vi "HEWH_WT300.vi"(4 "Manual Range (20 <10> A)":dbl(ring)=0.025 items=["5m <2.5m>"=0.0025, "10m <5m>"=0.005, "20m <10m>"=0.01, "50m <25m>"=0.025, "100m <50m>"=0.05, "200m <100m>"=0.1, "500m <250m>"=0.25, "1 <500m>"=0.5, "2 <1>"=1.0, "5 <2.5>"=2.5, "10 <5>"=5.0, "20 <10>"=10.0, "40 <20>"=20.0], 6 "Range Configuration (True)":bool[](array[boolean])=[FALSE, FALSE, FALSE, TRUE, FALSE, FALSE, FALSE, FALSE, FALSE, FALSE, FALSE, FALSE, FALSE], 8 "error in":errorcluster, 9 "Enable Auto Range (F: Disable)":bool, 11 "Message Queues out":T2) -> (0 "error out":errorcluster)   [LabVIEW 2023]
uses:
  Tenney/support/Message Queue/All Message Queues.ctl
  Tenney/support/Message Queue/Message Cluster.ctl
  Utility/Type Definitions/UTILITY Power Data.ctl
  Utility/Type Definitions/UTILITY Notifier.ctl
  FVIR and LDO/support/Message Queue/Enqueue Message (Single).vi
  FVIR and LDO/support/Message Queue/Message Queue.lvlib
  Drivers/Yokogawa WT300 Series/Yokogawa WT300 Series.lvlib
  Tenney/support/Message Queue/Tenney Message Queue.lvlib
panel:
  out "Loop Count":i32
  out "Power Data":T1={"Current (A):Element 1"=236.2, "Current (A):Element 2"=17.749, "Power (W):Sigma"=4192.0, "Watt Hours (Wh):Sigma"=0.0, "Voltage (V):Element 2"=236.2, "Voltage (V):Element 1"=236.2, "Current Crest Factor:Element 1"=0.0, "Current Crest Factor:Element 2"=0.0, "Voltage Harmonic (%):Element 1"=0.0, "Voltage Harmonic (%):Element 2"=0.0, "Voltage Crest Factor:Element 1"=0.0, "Voltage Crest Factor:Element 2"=0.0, "Time:Element 1"=0.0, "Frequency (Hz):Element 1"=0.0, "Apparent Power (VA):Element 1"=0.0, "Apparent Power (VA):Element 2"=0.0, "Power Factor:Element 1"=0.0, "Power Factor:Element 2"=0.0, "Max Watt Hours"=0.0, "Voltage (V):Element 2 Avg"=0.0, "Voltage (V):Element 1 Avg"=0.0} {"Voltage (V):Element 1 Avg" format="%.3g"; "Voltage (V):Element 2 Avg" format="%.3g"; "Max Watt Hours" format="%.3g"; "Power Factor:Element 2" format="%.3g"; "Power Factor:Element 1" format="%.3g"; "Apparent Power (VA):Element 2" format="%.3g"; "Apparent Power (VA):Element 1" format="%.3g"; "Frequency (Hz):Element 1" format="%.3g"; "Time:Element 1" format="%.3g"; "Voltage Crest Factor:Element 2" format="%.3g"; "Voltage Crest Factor:Element 1" format="%.3g"; "Voltage Harmonic (%):Element 2" format="%.3g"; "Voltage Harmonic (%):Element 1" format="%.3g"; "Current Crest Factor:Element 2" format="%.3g"; "Current Crest Factor:Element 1" format="%.3g"; "Voltage (V):Element 1" format="%.3g"; "Voltage (V):Element 2" format="%.3g"; "Watt Hours (Wh):Sigma" format="%.3f"; "Power (W):Sigma" format="%.3g"; "Current (A):Element 2" format="%.3e"; "Current (A):Element 1" format="%.3e"}
  out "Header File":string[][](array[string])=[["Instrument", "YOKOGAWA,WT332,C2QB17128V,F1.03\n"], ["Instr Driver Revision", "1.0 F1.03"], ["Start Time", "1.0"], ["Voltage Range", "6/1/2015 11:50 AM"], ["Current Range", "Auto"], ["Update Rate", "Auto"], ["Standard", "0.250"], ["Algorithm", "IEC62301 Ed.2(Auto)"], ["Stop Factor", "Linear Regression"], ["Valid Period", ""], ["Start Total Harmonic Distortion Uthd 1", "0.065"], ["Start Total Harmonic Distortion Uthd 2", ""], ["End Total Harmonic Distortion Uthd 1", ""], ["End Total Harmonic Distortion Uthd 2", ""], ["Max Power (Watts)", ""], ["Power Variation (%)", ""], ["", ""]]
  in  "Debug":bool
  out "Debug":string[](array[string])
  # "5m <2.5m> A"
  # "10m <5m> A"
  # "20m <10m> A"
  # "50m <25m> A"
  # "100m <50m> A"
  # "200m <100m> A"
  # "500m <250m> A"
  # "1 <500m> A"
  # "2 <1> A"
  # "5 <2.5> A"
  # "10 <5> A"
  # "20 <10> A"
  # "40 <20> A"
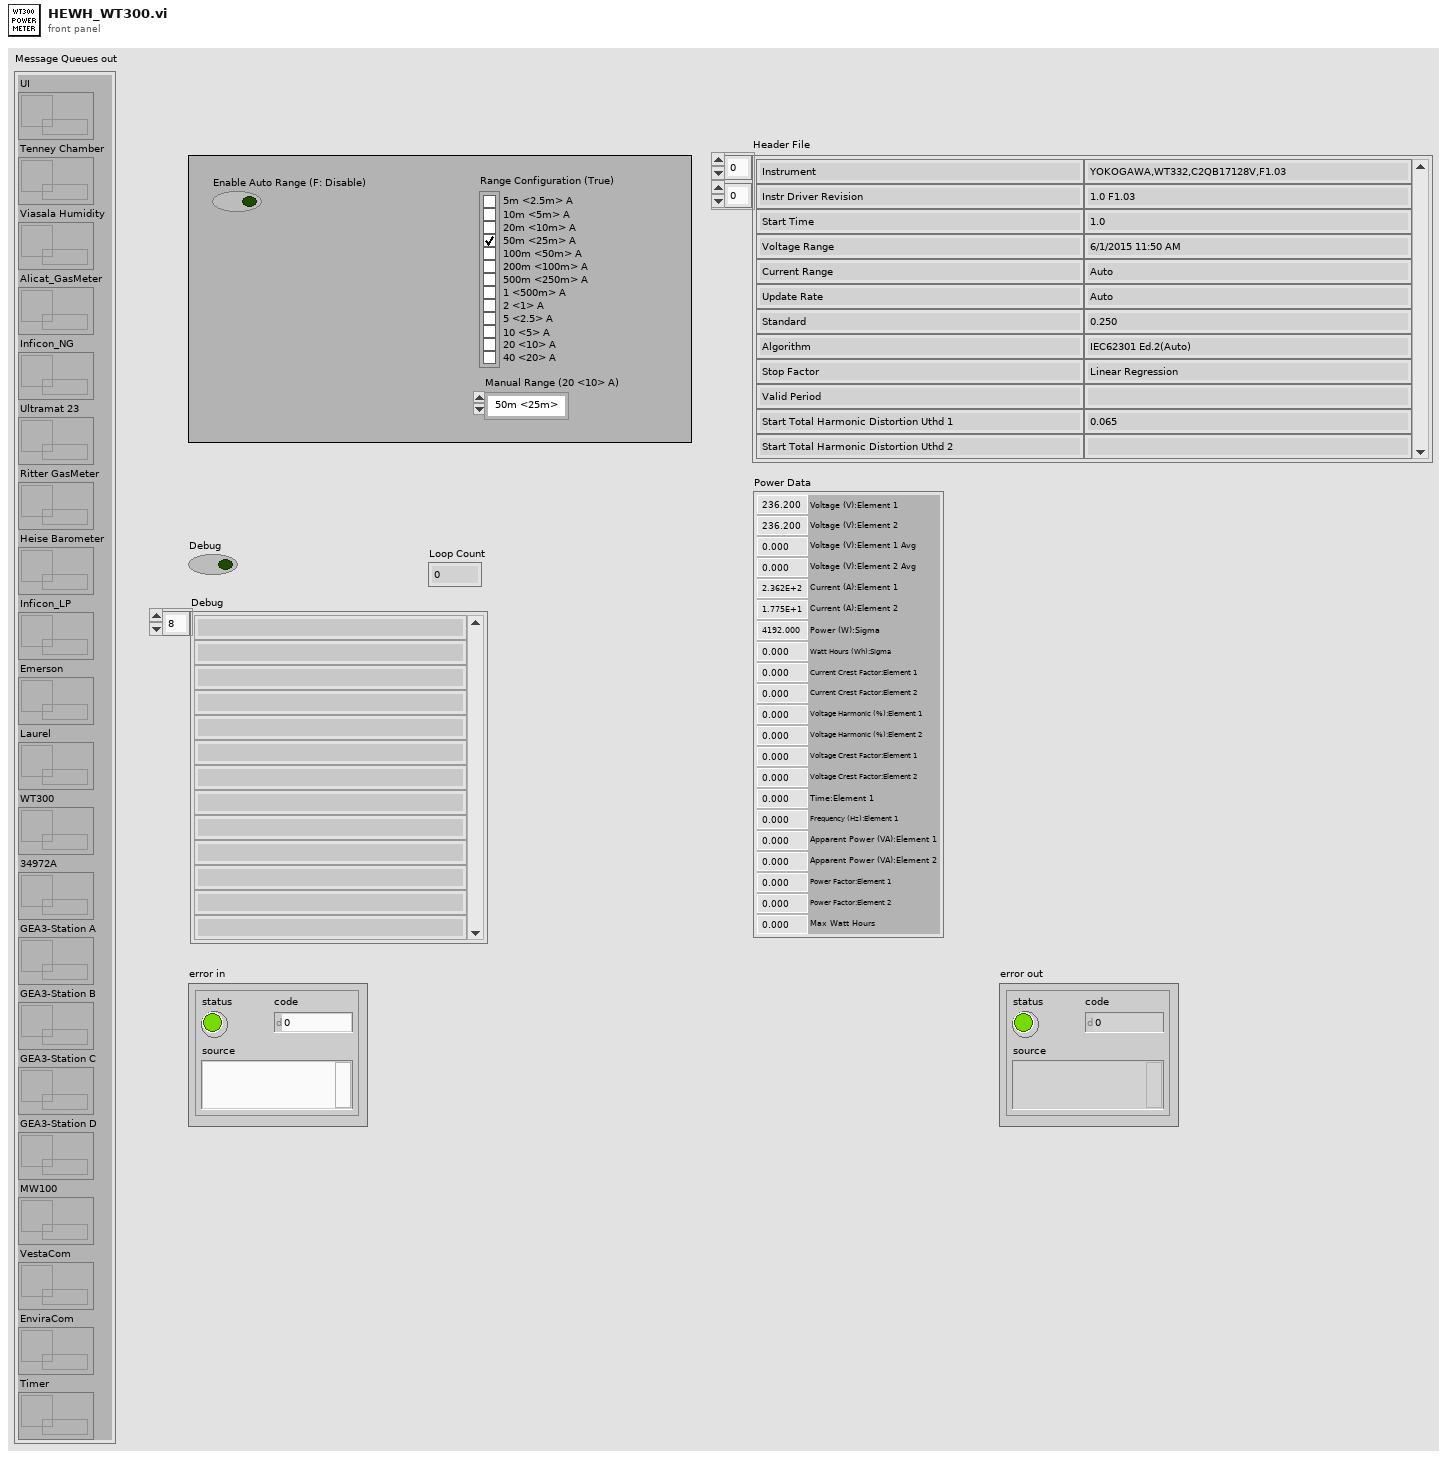
[diagram p1: front panel]
types:
  T1 = typedef "UTILITY Power Data.ctl" = cluster{"Current (A):Element 1":dbl, "Current (A):Element 2":dbl, "Power (W):Sigma":dbl, "Watt Hours (Wh):Sigma":dbl, "Voltage (V):Element 2":dbl, "Voltage (V):Element 1":dbl, "Current Crest Factor:Element 1":dbl, "Current Crest Factor:Element 2":dbl, "Voltage Harmonic (%):Element 1":dbl, "Voltage Harmonic (%):Element 2":dbl, "Voltage Crest Factor:Element 1":dbl, "Voltage Crest Factor:Element 2":dbl, "Time:Element 1":dbl, "Frequency (Hz):Element 1":dbl, "Apparent Power (VA):Element 1":dbl, "Apparent Power (VA):Element 2":dbl, "Power Factor:Element 1":dbl, "Power Factor:Element 2":dbl, "Max Watt Hours":dbl, "Voltage (V):Element 2 Avg":dbl, "Voltage (V):Element 1 Avg":dbl}
  T2 = typedef "Tenney Message Queue.lvlib/All Message Queues.ctl" = cluster{"UI":refnum<queue>, "Tenney Chamber":refnum<queue>, "Viasala Humidity":refnum<queue>, "Alicat_GasMeter":refnum<queue>, "Inficon_NG":refnum<queue>, "Ultramat 23":refnum<queue>, "Ritter GasMeter":refnum<queue>, "Heise Barometer":refnum<queue>, "Inficon_LP":refnum<queue>, "Emerson":refnum<queue>, "Laurel":refnum<queue>, "WT300":refnum<queue>, "34972A":refnum<queue>, "GEA3-Station A":refnum<queue>, "GEA3-Station B":refnum<queue>, "GEA3-Station C":refnum<queue>, "GEA3-Station D":refnum<queue>, "MW100":refnum<queue>, "VestaCom":refnum<queue>, "EnviraCom":refnum<queue>, "Timer":refnum<queue>}
  T3 = typedef "UTILITY Notifier.ctl" = enum16{"Set", "Read", "Release Ref"}
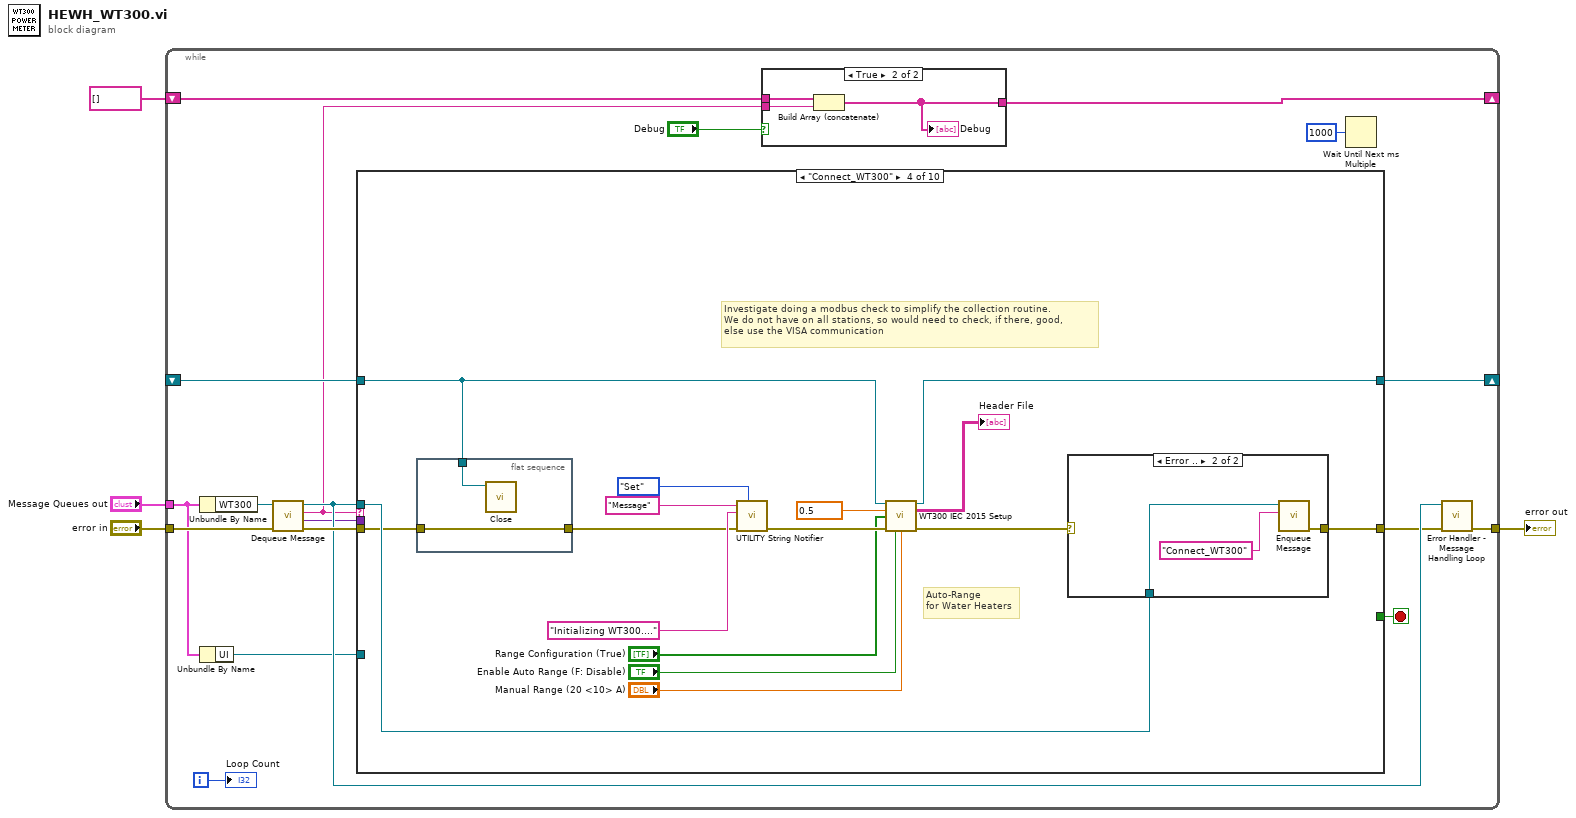
[diagram p0: block diagram]
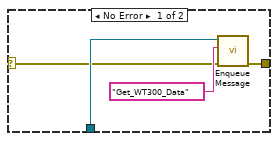
[diagram p6: hidden frame]
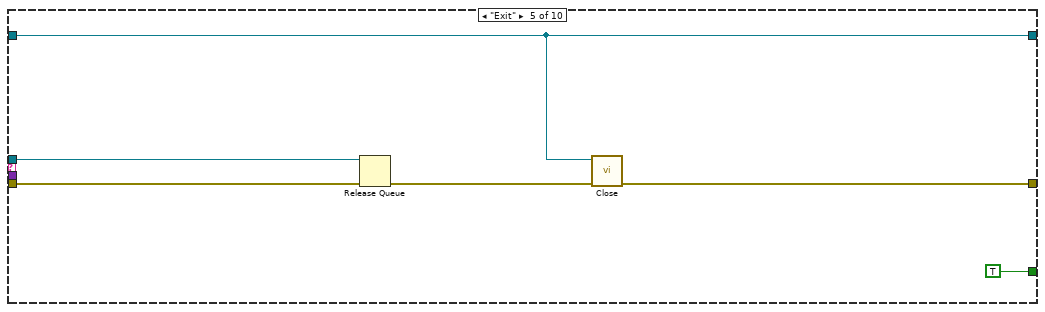
[diagram p7: hidden frame]
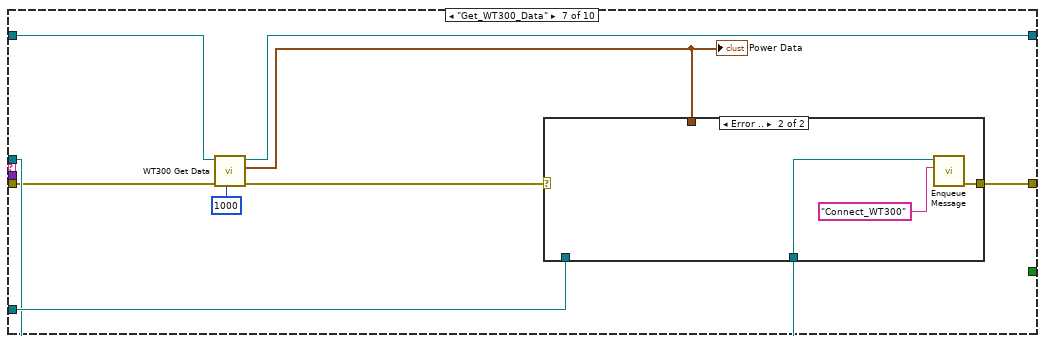
[diagram p9: hidden frame]
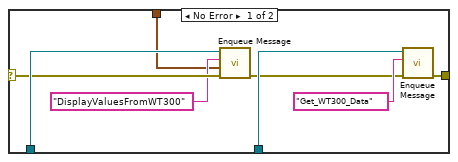
[diagram p10: hidden frame]
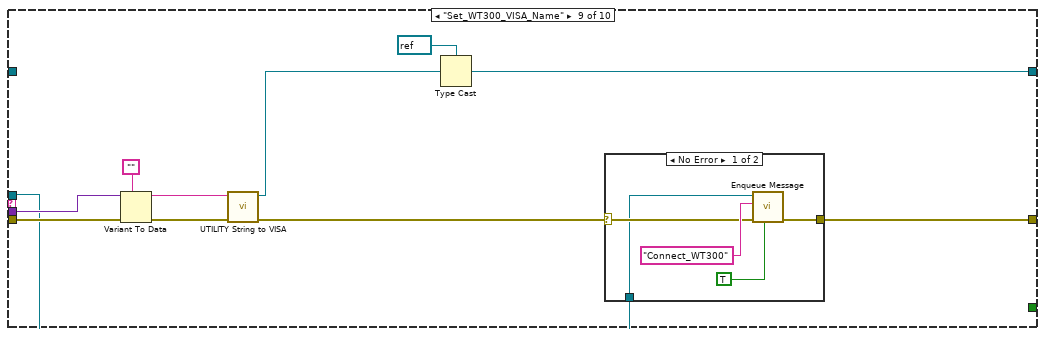
[diagram p12: hidden frame]
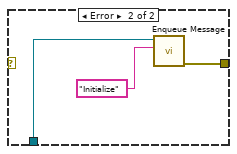
[diagram p13: hidden frame]
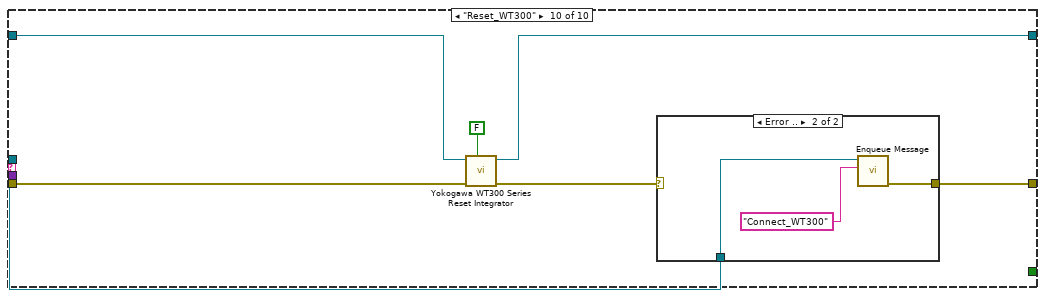
[diagram p14: hidden frame]
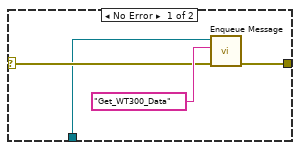
[diagram p15: hidden frame]
diagram:
  n1 = while {
    tunnel: "Message Queues out" -> [w12]
    tunnel: "error in" -> [w21]
    tunnel: [w17] -> w3
    shift-right: [w15] -> _
    shift-left: _ -> [w14]
    shift-right: [w8] -> _
    shift-left: string[] [] -> [w9]
    i -> [w5]
    stop <- w19 stop-if-true
    n2 = Unbundle By Name(w12) -> ("WT300"=w22:refnum<queue>)
    n3 = Unbundle By Name(w12) -> ("UI"=w11:refnum<queue>)
    n4 = call "Dequeue Message.vi"("error in (no error)"=w21, "Message Queue"=w22) -> ("error out"=w20:errorcluster, "Message Data"=w6:variant, "Message"=w10:string, "dup Message Queue"=w18:refnum<queue>)  [unwired: 6 in]
    n5 = case shown="\"Connect_WT300\"" w10 {
      tunnel: w20 -> [w27 w29 w31 w35 w61 w64 w69 w86 w95 w110]
      tunnel: [w27 w29 w31 w48 w59 w64 w73 w86 w92 w113] -> w16
      tunnel: [_ _ _ _ TRUE _ _ _ _ _] -> w19
      tunnel: w18 -> [_ _ _ w47 w62 _ w72 _ w91 w112]
      tunnel: [w28 w30 w32 w40 w58 w65 w67 w87 w88 w107] -> w15
      tunnel: w14 -> [w28 w30 w32 w33 w58 w65 w71 w87 _ w108]
      tunnel: w11 -> [_ _ _ _ _ _ w74 _ _ _]
      tunnel: w6 -> [_ _ _ _ _ _ _ _ w94 _]
      frame "---------- Setup ----------" {
      }
      frame Default {
      }
      frame "Initialize" {
      }
      frame "Connect_WT300" {
        w46 = 0.5 items=["100m"=0.1, "250m"=0.25, "500m"=0.5, "1"=1.0, "2"=2.0, "5"=5.0] ("Update Rate (250m s)")
        # "Investigate doing a modbus check to simplify the collection routine. \nWe do not have on all stations, so would need to check, if there, good, \nelse use the VISA communication"
        # "Auto-Range\nfor Water Heaters"
        n6 = flat-sequence {
          tunnel: w35 -> [w50]
          tunnel: [w50] -> w34
          tunnel: w33 -> [w49]
          frame #0 {
            n7 = call "Close.vi"("VISA resource name"=w49) -> ()  [unwired: 10 in, 1 out]
          }
        }
        n8 = call "UTILITY String Notifier.vi"("Status"=UTILITY_Notifier."Set", "error in (no error)"=w34, "Set Status"="Initializing WT300....", "name (unnamed)"="Message") -> ("error out"=w44:errorcluster)  [unwired: 6 in, 1 out]
        n9 = call "WT300 IEC 2015 Setup.vi"("VISA Input"=w33, "Update Rate (250m s)"=w46, "Range Configuration (True)"="Range Configuration (True)", "error in (no error)"=w44, "Enable Auto Range (F: Disable)"="Enable Auto Range (F: Disable)", "Manual Range (20 <10> A)"="Manual Range (20 <10> A)") -> ("VISA Output"=w40:refnum<visa-resource-name>, "Header File"=→"Header File":string[][], "error out"=w41:errorcluster)  [unwired: 7 in]
        n10 = case shown="Error .." w41 {
          selector: w41 -> [w51 _]
          tunnel: [w53 w56] -> w48
          tunnel: w47 -> [w52 w55]
          frame No Error {
            n11 = call-poly "Enqueue Message.vi"("error in (no error)"=w51, "Message"="Get_WT300_Data", "Message Queue"=w52) -> ("error out"=w53:errorcluster)  [unwired: 7 in, 1 out]
          }
          frame Error {
            n12 = call-poly "Enqueue Message.vi"("Message"="Connect_WT300", "Message Queue"=w55) -> ("error out"=w56:errorcluster)  [unwired: 8 in, 1 out]
          }
        }
      }
      frame "Exit" {
        n13 = Release Queue(queue=w62, error in (no error)=w61) -> (error out=w60:errorcluster)  [unwired: 1 in, 2 out]
        n14 = call "Close.vi"("error in (no error)"=w60, "VISA resource name"=w58) -> ("error out"=w59:errorcluster)  [unwired: 9 in]
      }
      frame "---------- Data Collection ----------" {
      }
      frame "Get_WT300_Data" {
        n15 = call "WT300 Get Data.vi"("Timeout (10000 ms)"=1000, "error in (no error)"=w69, "VISA resource name"=w71) -> ("error out"=w68:errorcluster, "Power Data"=w66:T1, "VISA resource name out"=w67:refnum<visa-resource-name>)  [unwired: 3 in, 3 out]
        "Power Data" <- w66
        n16 = case shown="Error .." w68 {
          selector: w68 -> [w77 _]
          tunnel: w74 -> [w82 _]
          tunnel: [w81 w84] -> w73
          tunnel: w72 -> [w80 w83]
          tunnel: w66 -> [w75 _]
          frame No Error {
            n17 = call-poly "Enqueue Message.vi"("error in (no error)"=w77, "Message Data"=w75, "Message"="DisplayValuesFromWT300", "Message Queue"=w82) -> ("error out"=w78:errorcluster)  [unwired: 6 in, 1 out]
            n18 = call-poly "Enqueue Message.vi"("error in (no error)"=w78, "Message"="Get_WT300_Data", "Message Queue"=w80) -> ("error out"=w81:errorcluster)  [unwired: 7 in, 1 out]
          }
          frame Error {
            n19 = call-poly "Enqueue Message.vi"("Message"="Connect_WT300", "Message Queue"=w83) -> ("error out"=w84:errorcluster)  [unwired: 8 in, 1 out]
          }
        }
      }
      frame "---------- Events ----------" {
      }
      frame "Set_WT300_VISA_Name" {
        n20 = Variant To Data(error in=w95, type="", Variant=w94) -> (data=w98:string, error out=w97:errorcluster)
        n21 = call "UTILITY String to VISA.vi"("error in (no error)"=w97, "VISA Name"=w98) -> ("error out"=w93:errorcluster, "VISA resource name out"=w90:refnum<visa-resource-name>)  [unwired: 8 in]
        n22 = Type Cast(type=refnum<visa-resource-name> refnum ("VISA resource name out"), x=w90) -> (*(type *) &x=w88:refnum<visa-resource-name>)
        n23 = case shown="No Error" w93 {
          selector: w93 -> [w101 _]
          tunnel: [w100 w105] -> w92
          tunnel: w91 -> [w99 w104]
          frame No Error {
            n24 = call-poly "Enqueue Message.vi"("Priority Message? (F)"=TRUE, "error in (no error)"=w101, "Message"="Connect_WT300", "Message Queue"=w99) -> ("error out"=w100:errorcluster)  [unwired: 6 in, 1 out]
          }
          frame Error {
            n25 = call-poly "Enqueue Message.vi"("Message"="Initialize", "Message Queue"=w104) -> ("error out"=w105:errorcluster)  [unwired: 8 in, 1 out]
          }
        }
      }
      frame "Reset_WT300" {
        n26 = call "Yokogawa WT300 Series Reset Integrator.vi"("Initialization Routing?"=FALSE, "Error In"=w110, "VISA Refnum in"=w108) -> ("Error Out"=w109:errorcluster, "VISA resource name out"=w107:refnum<visa-resource-name>)  [unwired: 7 in]
        n27 = case shown="Error .." w109 {
          selector: w109 -> [w116 _]
          tunnel: [w115 w119] -> w113
          tunnel: w112 -> [w114 w118]
          frame No Error {
            n28 = call-poly "Enqueue Message.vi"("error in (no error)"=w116, "Message"="Get_WT300_Data", "Message Queue"=w114) -> ("error out"=w115:errorcluster)  [unwired: 7 in, 1 out]
          }
          frame Error {
            n29 = call-poly "Enqueue Message.vi"("Message"="Connect_WT300", "Message Queue"=w118) -> ("error out"=w119:errorcluster)  [unwired: 8 in, 1 out]
          }
        }
      }
    }
    n30 = case shown="True" "Debug" {
      tunnel: w10 -> [_ w26]
      tunnel: w9 -> [w23 w25]
      tunnel: [w23 w24] -> w8
      frame False {
      }
      frame True {
        n31 = Build Array (concatenate)(w25, w26) -> (w24:string[])
        "Debug" <- w24
      }
    }
    n32 = Wait Until Next ms Multiple(millisecond multiple=u32 1000) -> ()  [unwired: 1 out]
    n33 = call "Error Handler - Message Handling Loop.vi"("error in (no error)"=w16, "Message Queue"=w18) -> ("dup error in"=w17:errorcluster)  [unwired: 8 in, 1 out]
    "Loop Count" <- w5
  }
  "error out" <- w3
